vi "to string array 1.0.vi"(8 "error in (no error)":errorcluster, 11 "Multiplexer configuration in":refnum<class "Multiplexer configuration.lvclass">) -> (0 "error out":errorcluster, 2 "Array":string[][](array[string]), 3 "Multiplexer configuration out":refnum<class "Multiplexer configuration.lvclass">)   [LabVIEW 2021, in "Multiplexer configuration.lvclass"]
uses:
  Multiplexer configuration.lvclass
  Multiplexer configuration.lvclass/Multiplexer configuration.ctl
  <vilib>/NI/Tag Bus Module Framework/channel/TBM channel.lvclass/TBM channel.ctl
  <vilib>/NI/Tag Bus/tag/tag descriptor.lvclass/tag descriptor.ctl
  Read Lines.vi
  <vilib>/NI/Tag Bus Module Framework/channel/TBM channel.lvclass
  C:/Program Files (x86)/National Instruments/LabVIEW 2021/vi.lib/NI/Tag Bus/tag/tag descriptor.lvclass
  <vilib>/NI/Tag Bus/tag/tag descriptor.lvclass
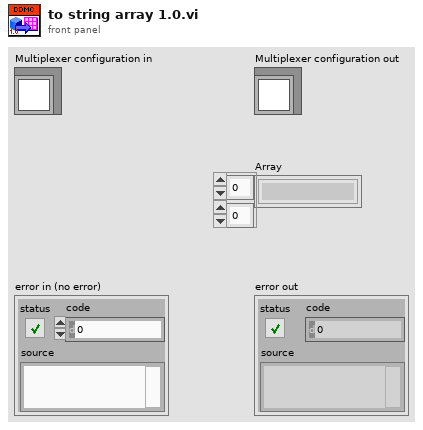
[diagram p1: front panel]
types:
  T1 = typedef "Multiplexer configuration.lvclass/Line.ctl" = cluster{"A":refnum<class "TBM channel.lvclass">, "B":refnum<class "TBM channel.lvclass">, "Select":refnum<class "TBM channel.lvclass">, "Output":refnum<class "TBM channel.lvclass">}
  T2 = typedef "TBM channel.lvclass/channel classification.ctl" = enum16{"input data", "output data", "processing parameter", "processing result"}
  T3 = typedef "tag bus.lvlib/tag descriptor.lvclass/Data Type.ctl" = enum16{"Double", "Single", "I64", "I32", "I16", "I8", "U64", "U32", "U16", "U8", "Boolean", "String", "Array of Double", "Array of Single", "Array of I64", "Array of I32", "Array of I16", "Array of I8", "Array of U64", "Array of U32", "Array of U16", "Array of U8", "Array of Boolean", "Array of String"}
  T4 = typedef "Multiplexer configuration.lvclass/permissions.ctl" = enum32{"Read from HW", "Write to HW"}
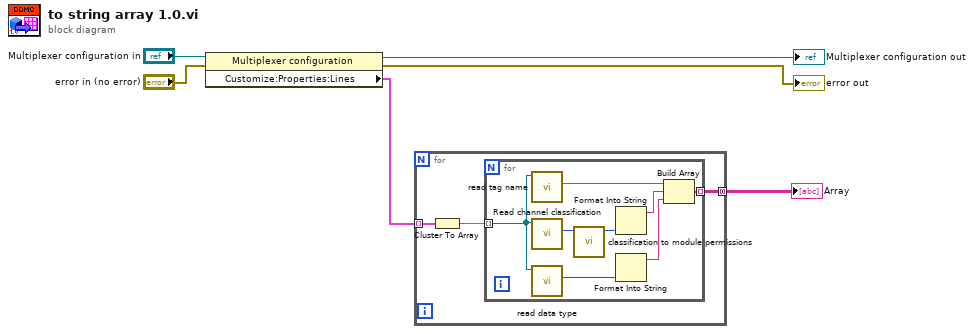
[diagram p0: block diagram]
diagram:
  n1 = property class="Multiplexer configuration"(reference="Multiplexer configuration in", error in="error in (no error)") -> (reference out=→"Multiplexer configuration out":refnum<class "Multiplexer configuration.lvclass">, error out=→"error out":errorcluster, "Customize:Properties:Lines"=w3:T1[])
  n2 = for {
    tunnel: w3 -> [w9] mode=indexing
    tunnel: [w7] -> w6 mode=concatenating
    n3 = Cluster To Array(cluster=w9) -> (array=w8:refnum<class "TBM channel.lvclass">[])
    n4 = for {
      tunnel: w8 -> [w13] mode=indexing
      tunnel: [w10] -> w7 mode=indexing
      n5 = call <vilib>:"read tag name.vi"("system tag in"=w13) -> ("name"=w17:string)  [unwired: 8 in, 2 out]
      n6 = call <vilib>:"Read channel classification.vi"("channel in"=w13) -> ("channel classification"=w16:T2)  [unwired: 8 in, 2 out]
      n7 = call <vilib>:"read data type.vi"("system tag in"=w13) -> ("data type"=w12:T3)  [unwired: 8 in, 2 out]
      n8 = call "classification to module permissions.vi"("channel classification"=w16) -> ("permissions"=w15:T4)  [unwired: 10 in]
      n9 = Format Into String(w15) -> (resulting string=w14:string)  [unwired: 3 in, 1 out]
      n10 = Format Into String(w12) -> (resulting string=w11:string)  [unwired: 3 in, 1 out]
      n11 = Build Array(w17, w14, w11) -> (w10:string[])
    }
  }
  "Array" <- w6
